vi "ex1.vi"() -> ()   [LabVIEW 2022 SP3]
panel:
  out "output value":dbl
  in  "Reset":bool
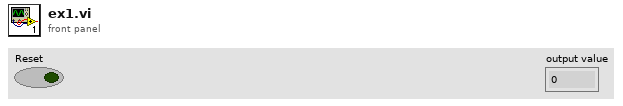
[diagram p1: front panel]
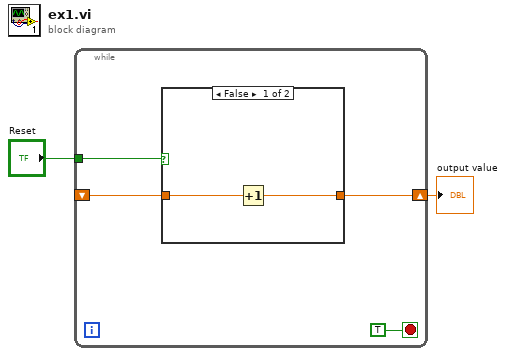
[diagram p0: block diagram]
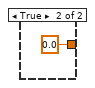
[diagram p2: hidden frame]
diagram:
  n1 = while {
    tunnel: "Reset" -> [w6]
    shift-right: [w4] -> w1
    shift-left: _ -> [w5]
    stop <- TRUE stop-if-true
    n2 = case shown="False" w6 {
      tunnel: w5 -> [w8 _]
      tunnel: [w7 0.0] -> w4
      frame False {
        n3 = Increment(x=w8) -> (x+1=w7:dbl)
      }
      frame True {
      }
    }
  }
  "output value" <- w1
